vi "_CommandInfo.vi"() -> (0 "command info":T1)   [LabVIEW 2014, in "tango.lvlib"]
uses:
  tango.lvlib
panel:
  # "CommandInfo.level\n-----------------------\n\tOPERATOR = 0\n EXPERT = 1"
  # "CommandInfo.in-out-type\n-----------------------\n\tDEV_VOID = 0\n\tDEV_BOOLEAN = 1\n\tDEV_SHORT = 2\n\tDEV_LONG = 3\n\tDEV_FLOAT = 4\n\tDEV_DOUBLE = 5\n\tDEV_USHORT = 6\n\tDEV_ULONG = 7\n\tDEV_STRING = 8\n\tDEVVAR_CHARARRAY = 9\n\tDEVVAR_SHORTARRAY = 10\n\tDEVVAR_LONGARRAY = 11\n\tDEVVAR_FLOATARRAY = 12\n\tDEVVAR_DOUBLEARRAY = 13\n\tDEVVAR_USHORTARRAY = 14\n\tDEVVAR_ULONGARRAY = 15\n\tDEVVAR_STRINGARRAY = 16\n\tDEVVAR_LONGSTRINGARRAY = 17\n\tDEVVAR_DOUBLESTRINGARRAY = 18\n\tDEV_STATE = 19\n\tCONST_DEV_STRING = 20\n\tDEVVAR_BOOLEANARRAY = 21\n\tDEV_UCHAR = 22\n\tDEV_LONG64 = 23\n\tDEV_ULONG64 = 24\n\tDEVVAR_LONG64ARRAY = 25\n\tDEVVAR_ULONG64ARRAY = 26\n\tDEV_INT = 26\n\tDEV_ENCODED = 28"
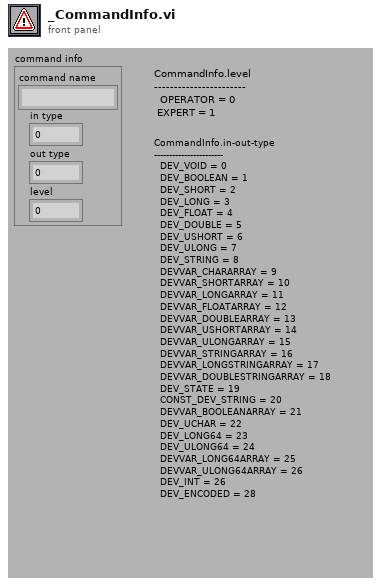
[diagram p1: front panel]
types:
  T1 = cluster{"command name":string, "in type":i16, "out type":i16, "level":i16}
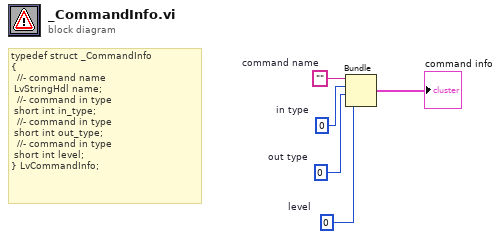
[diagram p0: block diagram]
diagram:
  w2 = i16 0  # level
  w3 = ""  # command name
  w4 = i16 0  # out type
  w5 = i16 0  # in type
  # "typedef struct _CommandInfo\n{\n  //- command name\n\tLvStringHdl name;\n  //- command in type\n\tshort int in_type;\n  //- command in type\n\tshort int out_type;\n  //- command in type\n\tshort int level;\n} LvCommandInfo;"
  n1 = Bundle("command name"=w3, "in type"=w5, "out type"=w4, "level"=w2) -> (→"command info":T1)  [unwired: 1 in]
